vi "Exp_ICCD_GetSequentialStartingGateProperties.vi"(8 "error in (no error)":errorcluster, 11 "LightField Automation in":refnum<class "LightField Automation.lvclass">) -> (0 "error out":errorcluster, 1 "Sequential Starting Gate Width (ns)":dbl, 2 "Sequential Starting Gate Delay (ns)":dbl, 3 "LightField Automation out":refnum<class "LightField Automation.lvclass">)   [LabVIEW 2020, in "LightField Automation.lvclass"]
uses:
  LightField Automation.lvclass
  C:/Program Files/Princeton Instruments/LightField/PrincetonInstruments.LightFieldAddInSupportServices.dll
  C:/Program Files/Princeton Instruments/LightField/AddInViews/PrincetonInstruments.LightFieldViewV3.dll
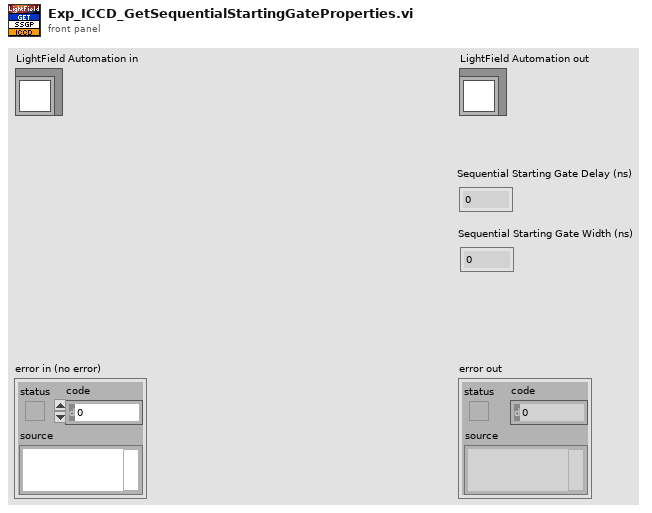
[diagram p1: front panel]
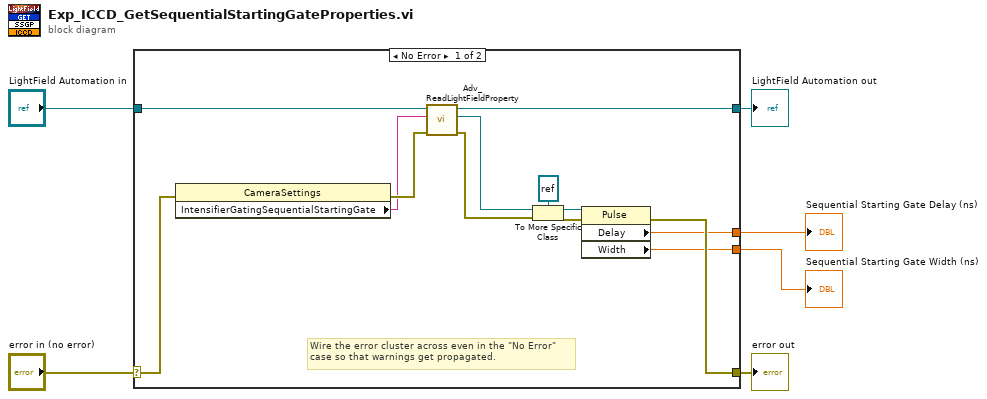
[diagram p0: block diagram]
diagram:
  n1 = case shown="No Error" "error in (no error)" {
    selector: "error in (no error)" -> [w19 w21]
    tunnel: [w15 w21] -> w5
    tunnel: [w11 w20] -> w3
    tunnel: "LightField Automation in" -> [w12 w20]
    tunnel: [w14 _] -> w2
    tunnel: [w13 _] -> w1
    frame No Error {
      # "Wire the error cluster across even in the \"No Error\"\ncase so that warnings get propagated."
      n2 = property class="CameraSettings"(error in=w19) -> (error out=w10:errorcluster, "IntensifierGatingSequentialStartingGate"=w9:string)  [unwired: 1 in, 1 out]
      n3 = call "Adv_ReadLightFieldProperty.vi"("error in (no error)"=w10, "setting"=w9, "LightField Automation in"=w12) -> ("error out"=w8:errorcluster, "value"=w7:refnum<k24>, "LightField Automation out"=w11:refnum<class "LightField Automation.lvclass">)  [unwired: 6 in]
      n4 = To More Specific Class(target class=refnum<k24> refnum ("reference out"), reference=w7, error in=w8) -> (specific class reference=w17:refnum<k24>, error out=w16:errorcluster)
      n5 = property class="Pulse"(reference=w17, error in=w16) -> (error out=w15:errorcluster, "Delay"=w14:dbl, "Width"=w13:dbl)  [unwired: 1 out]
    }
    frame Error {
    }
  }
  "error out" <- w5
  "LightField Automation out" <- w3
  "Sequential Starting Gate Delay (ns)" <- w2
  "Sequential Starting Gate Width (ns)" <- w1
